vi "Write T ctl driver.vi"(8 "error in (no error)":errorcluster, 10 "Temperature Controller Driver.lvclass":refnum<class "Temperature Controller Driver.lvclass">, 11 "Temperature Controller in":refnum<class "Temperature Controller.lvclass">) -> (0 "error out":errorcluster, 3 "Temperature Controller out":refnum<class "Temperature Controller.lvclass">)   [LabVIEW 2018, in "Temperature Controller.lvclass"]
uses:
  Temperature Controller.lvclass
  C:/github/2018/LabActor/Instrument Actor/Instrument Actor.lvclass
  NHMFL_Core/Libraries/Instruments/Temperature Controller Driver/Temperature Controller Driver.lvclass
  C:/github/2018/NHMFL_Core/Libraries/Instruments/Instrument Driver/Instrument Driver.lvclass
  Instrument Actor/Instrument Actor.lvclass/Instrument Actor.ctl
  Instrument Actor/Write Instrument driver.vi
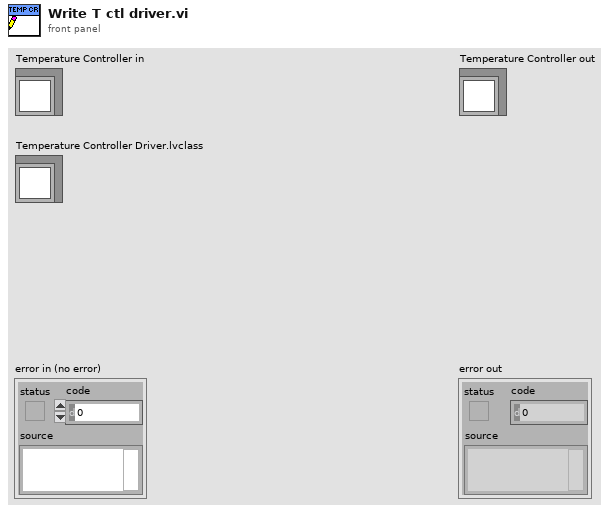
[diagram p1: front panel]
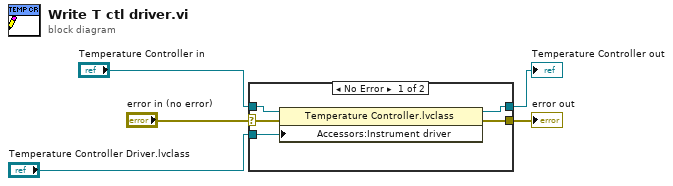
[diagram p0: block diagram]
diagram:
  n1 = case shown="No Error" "error in (no error)" {
    selector: "error in (no error)" -> [w7 w11]
    tunnel: [w6 w11] -> w4
    tunnel: [w9 w12] -> w2
    tunnel: "Temperature Controller in" -> [w10 w12]
    tunnel: "Temperature Controller Driver.lvclass" -> [w8 _]
    frame No Error {
      n2 = property class="Temperature Controller.lvclass"(reference=w10, error in=w7, "Accessors:Instrument driver"=w8) -> (reference out=w9:refnum<class "Temperature Controller.lvclass">, error out=w6:errorcluster)
    }
    frame Error {
    }
  }
  "error out" <- w4
  "Temperature Controller out" <- w2
